vi "Do Transition.vi"(6 "Actions In":refnum<class "Iteration Actions.lvclass">, 11 "State Transition in":refnum<class "State Transition.lvclass">) -> (3 "State Transition out":refnum<class "State Transition.lvclass">, 4 "Actions":refnum<class "Iteration Actions.lvclass">)   [LabVIEW 2020, in "VolatusSeq.lvlib" / "State Transition.lvclass"]
uses:
  State Transition.lvclass
  Iteration Actions/Iteration Actions.lvclass
  State Transition.lvclass/State Transition.ctl
  Iteration Actions/Iteration Actions.lvclass/Iteration Actions.ctl
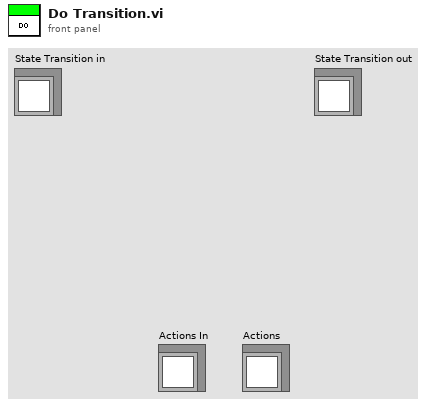
[diagram p1: front panel]
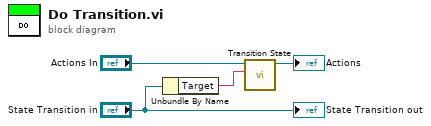
[diagram p0: block diagram]
diagram:
  n1 = Unbundle By Name("State Transition in") -> ("Target"=w1:string)
  n2 = call "Transition State.vi"("Next State"=w1, "Iteration Actions in"="Actions In") -> ("Iteration Actions out"=→"Actions":refnum<class "Iteration Actions.lvclass">)  [unwired: 8 in, 1 out]
  "State Transition out" <- "State Transition in"
